vi "Created Aliases.vi"(11 "Actor in":refnum<class "Actor.lvclass">) -> (2 "Created Aliases":T1)   [LabVIEW 2021, in "jettl.lvlib" / "Actor.lvlib" / "Actor.lvclass"]
uses:
  Actor.lvclass
  Created Aliases.ctl
  Actor.lvlib
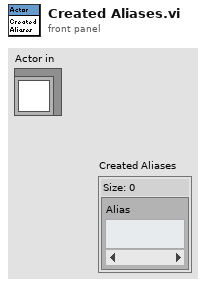
[diagram p1: front panel]
types:
  T1 = typedef "jettl.lvlib/Actor.lvlib/Created Aliases.ctl" = set{string}
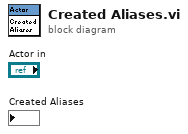
[diagram p0: block diagram]
diagram:
